vi "Trigger.vi"(9 "Trigger OUT":bool, 10 "Trigger IN":bool, 11 "Comport":refnum<visa-resource-name>) -> ()   [LabVIEW 2016]
uses:
  <vilib>/Instr/_visa.llb/VISA Configure Serial Port (Instr).vi
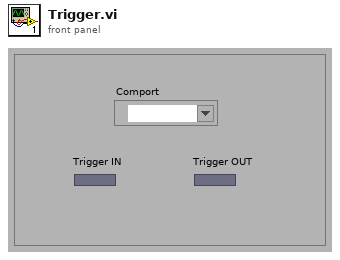
[diagram p1: front panel]
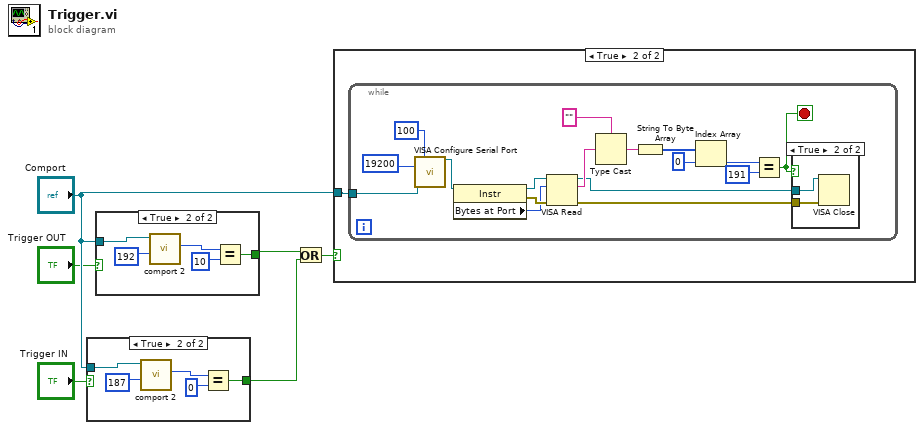
[diagram p0: block diagram]
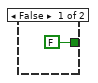
[diagram p4: hidden frame]
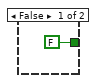
[diagram p5: hidden frame]
diagram:
  n1 = case shown="True" "Trigger IN" {
    tunnel: "Comport" -> [_ w9]
    tunnel: [FALSE w8] -> w6
    frame False {
    }
    frame True {
      n2 = call "comport 2.vi"("x"=187, "VISA resource name"=w9) -> ("Numeric"=w11:u8)  [unwired: 7 in, 2 out]
      n3 = Equal?(x=w11, y=u8 0) -> (x = y?=w8:bool)
    }
  }
  n4 = case shown="True" "Trigger OUT" {
    tunnel: "Comport" -> [_ w18]
    tunnel: [FALSE w14] -> w5
    frame False {
    }
    frame True {
      n5 = call "comport 2.vi"("x"=192, "VISA resource name"=w18) -> ("Numeric"=w16:u8)  [unwired: 7 in, 2 out]
      n6 = Equal?(x=w16, y=u8 10) -> (x = y?=w14:bool)
    }
  }
  n7 = Or(x=w5, y=w6) -> (x .or. y?=w4:bool)
  n8 = case shown="True" w4 {
    tunnel: "Comport" -> [_ w19]
    frame False {
    }
    frame True {
      n9 = while {
        tunnel: w19 -> [w23]
        stop <- w22 stop-if-true
        n10 = call-poly "VISA Configure Serial Port"("VISA resource name"=w23, "timeout (10sec)"=u32 100, "baud rate (9600)"=u32 19200) -> ("VISA resource name out"=w30:refnum<visa-resource-name>)  [unwired: 11 in, 1 out]
        n11 = property class="Instr"(reference=w30) -> (reference out=w26:refnum<visa-resource-name>, error out=w28:errorcluster, "Bytes at Port"=w27:u32)  [unwired: 1 in]
        n12 = VISA Read(VISA resource name=w26, byte count=w27, error in (no error)=w28) -> (VISA resource name out=w25:refnum<visa-resource-name>, read buffer=w35:string, error out=w29:errorcluster)  [unwired: 1 out]
        n13 = Type Cast(type="", x=w35) -> (*(type *) &x=w36:string)
        n14 = String To Byte Array(string=w36) -> (unsigned byte array=w34:u8[])
        n15 = Index Array(array=w34, index=0) -> (element=w32:u8)
        n16 = Equal?(x=w32, y=u8 191) -> (x = y?=w22:bool)
        n17 = case shown="True" w22 {
          tunnel: w25 -> [_ w38]
          tunnel: w29 -> [_ w37]
          frame False {
          }
          frame True {
            n18 = VISA Close(VISA resource name=w38, error in (no error)=w37) -> ()  [unwired: 1 out]
          }
        }
      }
    }
  }
